vi "calibration_loadcell.vi"() -> ()   [LabVIEW 2011]
uses:
  Instance           1 28Saved   Loadcell_Calibration .vi
panel:
  out "Waveform Graph":dynamicdata(graph)
  in  "file path (dialog if empty)":path
  in  "Numeric":i32=100
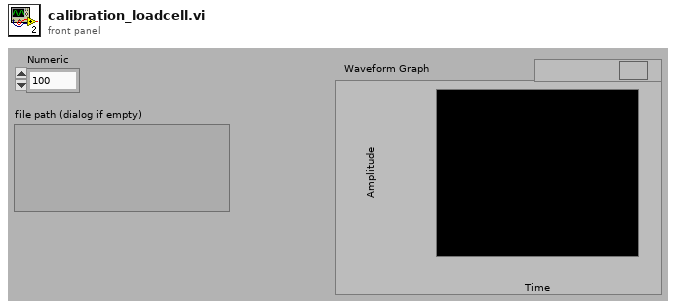
[diagram p1: front panel]
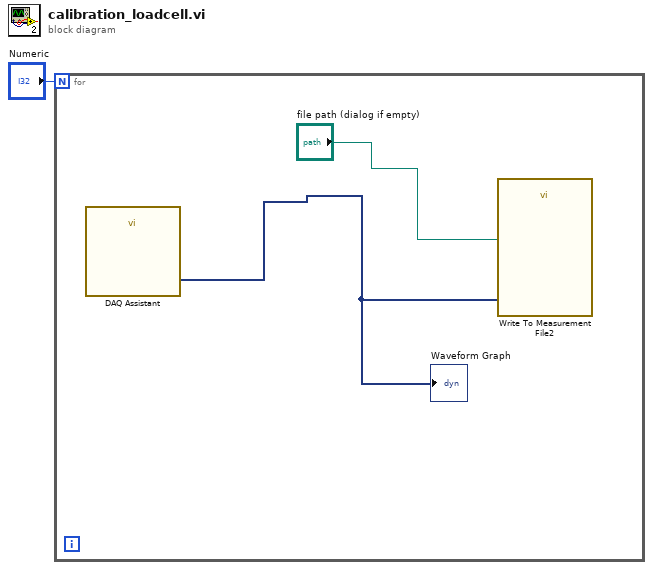
[diagram p0: block diagram]
diagram:
  n1 = for {
    N: "Numeric" -> [_]
    n2 = call "DAQ Assistant"() -> ("data"=w2:dynamicdata)  [unwired: 16 in, 3 out]
    "Waveform Graph" <- w2
    n3 = call "Write To Measurement File2"("Signals"=w2, "Filename"="file path (dialog if empty)") -> ()  [unwired: 15 in, 3 out]
  }
